vi "Init Core.vi"(7 "Environment Options (Defaults)":T1, 8 "error in (no error)":errorcluster, 10 "Path Overrides (Empty=Default)":T2 caption="Path Overrides", 11 "WebView2 Control in":refnum<class "WebView2 Control.lvclass">) -> (0 "error out":errorcluster, 3 "WebView2 Control out":refnum<class "WebView2 Control.lvclass">)   [LabVIEW 2020, in "WebView2.lvlib" / "WebView2 Control.lvclass"]
uses:
  WebView2 Control.lvclass
  Paths.ctl
  Core Env Options.ctl
  WebView2 Control.lvclass/WebView2 Control.ctl
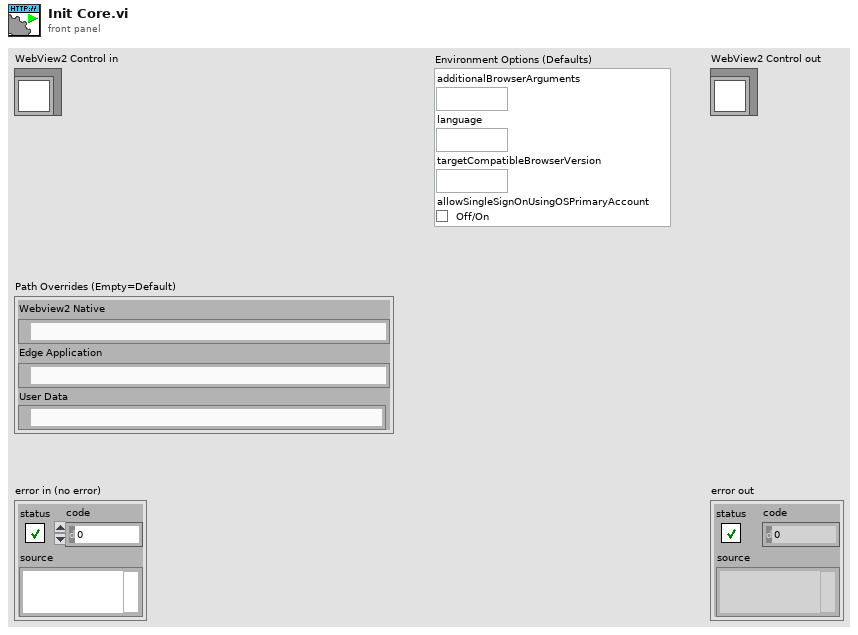
[diagram p1: front panel]
types:
  T1 = typedef "WebView2.lvlib/WebView2 Control.lvclass/Core Env Options.ctl" = cluster{"additionalBrowserArguments":string, "language":string, "targetCompatibleBrowserVersion":string, "allowSingleSignOnUsingOSPrimaryAccount":bool}
  T2 = typedef "WebView2.lvlib/WebView2 Control.lvclass/Paths.ctl" = cluster{"Webview2 Native":path, "Edge Application":path, "User Data":path}
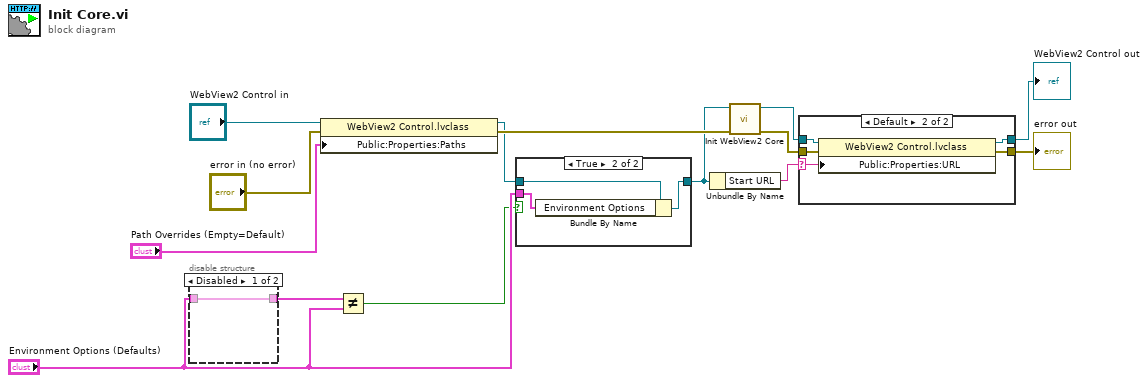
[diagram p0: block diagram]
diagram:
  n1 = disable-structure shown="Disabled" {
    disable-tunnel: [w15 _] -> w8
    disable-tunnel: "Environment Options (Defaults)" -> [w15 _]
    frame Disabled {
    }
    frame Enabled {
    }
  }
  n2 = property class="WebView2 Control.lvclass"(reference="WebView2 Control in", error in="error in (no error)", "Public:Properties:Paths"="Path Overrides (Empty=Default)") -> (reference out=w10:refnum<class "WebView2 Control.lvclass">, error out=w12:errorcluster)
  n3 = Not Equal?(x=w8, y="Environment Options (Defaults)") -> (x != y?=w6:bool)
  n4 = case shown="True" w6 {
    tunnel: [w16 w19] -> w2
    tunnel: w10 -> [w16 w18]
    tunnel: "Environment Options (Defaults)" -> [_ w17]
    frame False {
    }
    frame True {
      n5 = Bundle By Name(cluster=w18, "Environment Options"=w17) -> (w19:refnum<class "WebView2 Control.lvclass">)
    }
  }
  n6 = Unbundle By Name(w2) -> ("Start URL"=w1:string)
  n7 = call "Init WebView2 Core.vi"("error in (no error)"=w12, "WebView2"=w2) -> ("error out"=w13:errorcluster, "WebView2.lvlib:WebView2 Control.lvclass"=w4:refnum<class "WebView2 Control.lvclass">)  [unwired: 8 in]
  n8 = case shown="Default" w1 {
    selector: w1 -> [_ w22]
    tunnel: w13 -> [w20 w26]
    tunnel: [w20 w25] -> w5
    tunnel: w4 -> [w21 w24]
    tunnel: [w21 w23] -> w3
    frame "\u0000" {
    }
    frame Default {
      n9 = property class="WebView2 Control.lvclass"(reference=w24, error in=w26, "Public:Properties:URL"=w22) -> (reference out=w23:refnum<class "WebView2 Control.lvclass">, error out=w25:errorcluster)
    }
  }
  "error out" <- w5
  "WebView2 Control out" <- w3
